vi "AG34980A_Initialize.vi"(0 "VISA resource name":refnum<visa-resource-name>, 5 "ID Query (True)":bool=TRUE, 9 "Reset (True)":bool=TRUE, 11 "error in (no error)":errorcluster) -> (4 "VISA session":refnum<visa-resource-name>, 15 "error out":errorcluster)   [LabVIEW 2022 SP3, in "DMM_Keysight_34980A.lvlib" / "DMM_Keysight_34980A.lvclass"]
doc: "This VI initializes a connection with a 34980A instrument mainframe. You can optionally reset the instrument by setting the front panel reset control. You must run this VI before using any of the instrument driver VIs for this instrument."
uses:
  DMM_Keysight_34980A.lvclass
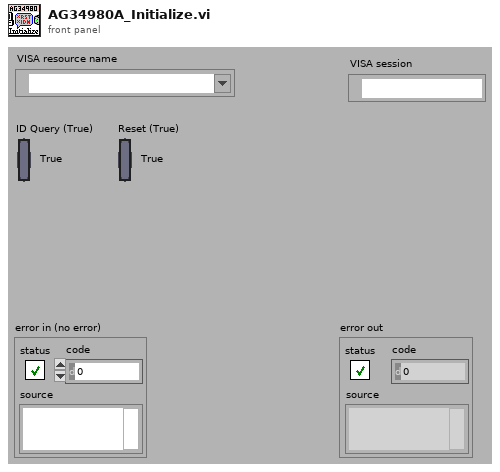
[diagram p1: front panel]
types:
  T1 = cluster{"status":bool, "code":i32, "VI Name":string}
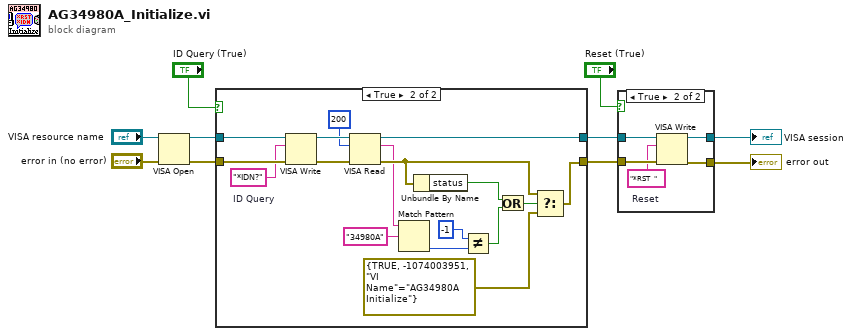
[diagram p0: block diagram]
diagram:
  n1 = VISA Open(error in (no error)="error in (no error)", VISA resource name="VISA resource name") -> (VISA resource name=w6:refnum<visa-resource-name>, error out=w8:errorcluster)  [unwired: 3 in]
  n2 = case shown="True" "ID Query (True)" {
    tunnel: [w11 w29] -> w4
    tunnel: [w12 w28] -> w5
    tunnel: w6 -> [w12 w17]
    tunnel: w8 -> [w11 w18]
    frame False {
    }
    frame True {
      w16 = "*IDN?"  # ID Query
      n3 = VISA Write(VISA resource name=w17, write buffer=w16, error in (no error)=w18) -> (VISA resource name out=w20:refnum<visa-resource-name>, error out=w22:errorcluster)  [unwired: 1 out]
      n4 = VISA Read(VISA resource name=w20, byte count=u32 200, error in (no error)=w22) -> (VISA resource name out=w28:refnum<visa-resource-name>, read buffer=w14:string, error out=w21:errorcluster)  [unwired: 1 out]
      n5 = Match Pattern(string=w14, regular expression="34980A") -> (offset past match=w27:i32)  [unwired: 1 in, 3 out]
      n6 = Unbundle By Name(w21) -> ("status"=w24:bool)
      n7 = Not Equal?(x=-1, y=w27) -> (x != y?=w19:bool)
      n8 = Or(x=w24, y=w19) -> (x .or. y?=w23:bool)
      n9 = Select(t=w21, s=w23, f=cluster{bool, i32, "VI Name":string} {TRUE, -1074003951, "VI Name"="AG34980A Initialize"}) -> (s? t:f=w29:T1)
    }
  }
  n10 = case shown="True" "Reset (True)" {
    tunnel: w5 -> [w31 w36]
    tunnel: w4 -> [w30 w33]
    tunnel: [w30 w34] -> w2
    tunnel: [w31 w35] -> w1
    frame False {
    }
    frame True {
      w32 = "*RST  "  # Reset
      n11 = VISA Write(VISA resource name=w36, write buffer=w32, error in (no error)=w33) -> (VISA resource name out=w35:refnum<visa-resource-name>, error out=w34:errorcluster)  [unwired: 1 out]
    }
  }
  "error out" <- w2
  "VISA session" <- w1
